vi "Update RefDAQ Parameters.vi"(0 "RefDAQParam":T1={"Full Frame Size"=0, "Ref Field of View"=0.0, "Ref Zoom"=0, "Ref_dwellTime"=0.0, "Ref X-pixels-per-line(Npxr)"=0, "Ref Y-lines-per-image(Npyr)"=0, "Ref Z-lines-per-image"=0, "Ignore Z lines"=0, "Ref Scan Cycles"=0, "Ref threshold XY"=0, "Ref threshold Z"=1, "Ref average XY"=1, "Ref Average  Z"=0, "Proportional_scale"=1.5999755859375, "Integral_scale"=2047.9375, "Proportional_scale Z"=1.5999755859375, "Integral_scale Z"=400.0, "Diff_threshold"=0.0, "Diff_threshold _z"=0.0, "Sliding Average"=FALSE, "Ref count reset enabled"=TRUE} caption="Reference frame DAQ setup" {"Proportional_scale Z" format="%#_15g"; "Ref average XY" min=1 max=64 step=1; "Diff_threshold" format="%#_15g"; "Diff_threshold _z" format="%#_15g"; "Proportional_scale" format="%#_15g"}, 11 "error in (no error)":errorcluster) -> (4 "Refnum out":T2, 15 "error out":errorcluster)   [LabVIEW 2020]
uses:
  RIG-SPECIFIC FILES/FPGA Refs/FPGA Ref.ctl
  Acquisition/Typedefs/Ref DAQ Param.ctl
  Typedefs/HW config states enum.ctl
  Global Variables/General Globals.vi
  Global Variables/gl_UI Ctrl Refs.vi
  <vilib>/Utility/error.llb/Error Cluster From Error Code.vi
  <vilib>/rvi/errors/niLvFpgaAdjustHostInterfaceError.vi
  <vilib>/rvi/interface/nirviReadWriteControl/nirviReadWriteControl.xnode
  NiFpgaLv.dll
  <vilib>/rvi/interface/Simulation/niFpgaSimulationCallBeginRW.vi
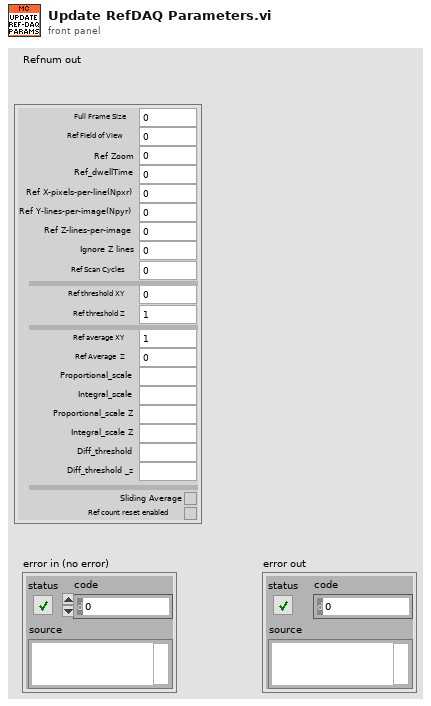
[diagram p1: front panel]
types:
  T1 = typedef "Ref DAQ Param.ctl" = cluster{"Full Frame Size":u16, "Ref Field of View":sgl, "Ref Zoom":i8, "Ref_dwellTime":sgl, "Ref X-pixels-per-line(Npxr)":i16, "Ref Y-lines-per-image(Npyr)":i16, "Ref Z-lines-per-image":i16, "Ignore Z lines":i16, "Ref Scan Cycles":i32, "Ref threshold XY":u16, "Ref threshold Z":u16, "Ref average XY":u16, "Ref Average  Z":u16, "Proportional_scale":fxp<+,16,2>, "Integral_scale":fxp<+/-,16,12>, "Proportional_scale Z":fxp<+,16,2>, "Integral_scale Z":fxp<+/-,16,12>, "Diff_threshold":fxp<+,16,2>, "Diff_threshold _z":fxp<+,16,2>, "Sliding Average":bool, "Ref count reset enabled":bool}
  T2 = typedef "FPGA Ref.ctl" = refnum<k20>
  T3 = typedef "HW config states enum.ctl" = enum16{"Load from file", "Save to file", "Save backup", "Write all", "Read all", "Write XY stage settings", "Write DAQ FPGA settings", "Write Control FPGA settings", "Write Phys Channels", "Write System Config", "Write HW Config", "Save System Config", "Save HW Config", "Clear", "Compare from file"}
  T4 = typedef "Hardware Configuration settings.ctl" = cluster{"Dev. PC":bool, "Swap XY on stage":bool, "No of AOD":u8, "MC Supported":bool, "Axial MC":bool, "Computer MAC address":string, "Externalise Triggers":bool, "Trigger HW config":T5, "DAQmx Chan":T6, "XY stage available":bool, "XY Stage":T7, "Z stage available":bool, "Z Stage config cluster":T8, "Encoder available":bool, "Encoder":T9, "VidRec available":bool, "Cam VidRec":T10, "Laser Power Control HW config":T11, "Laser 1 available":bool, "Laser 1 config cluster":T12, "Prechirper 1 available":bool, "Prechirper 1 config cluster":T13, "Control system.FPGA available?":bool, "Control Sys. HW config":T14, "DAQ FPGA HW Config":T15, "PMT Voltage Range":T18}
  T5 = typedef "Triggers HW config.ctl" = cluster{"Available Device List":i32, "Device Address":string}
  T6 = typedef "DAQmx physical channels cluster.ctl" = cluster{"Pockels AO":tag, "Hard shutter AO":tag, "PMT AOs":tag, "Galvo AOs":tag, "Power meter AI":tag}
  T7 = typedef "XY Stage config cluster.ctl" = cluster{"COM port":refnum<visa-resource-name>, "Baudrate":i32, "Type":string}
  T8 = typedef "Z Stage config cluster.ctl" = cluster{"COM port":refnum<visa-resource-name>, "Baudrate":i32, "Type":string}
  T9 = typedef "Encoder config cluster.ctl" = cluster{"IP address":string, "Port":u16, "Wheel radius (cm)":dbl, "Encoder Trigger":tag}
  T10 = typedef "Cam VidRec HW config setup cluster.ctl" = cluster{"DO flag-Video record":tag, "DO flag-Trial start":tag}
  T11 = typedef "Laser Power Control HW config.ctl" = cluster{"Laser Power Control":string, "Laser Power Modulation Control":enum16{"NI", "FPGA"}}
  T12 = typedef "Laser 1 config cluster.ctl" = cluster{"COM port":refnum<visa-resource-name>, "Baud Rate":i32, "Type":string}
  T13 = typedef "PreChirper 1 config cluster.ctl" = cluster{"Type":string, "Baud Rate":i32, "COM port":refnum<visa-resource-name>}
  T14 = typedef "Control Sys HW config cluster.ctl" = cluster{"Control system.FPGA Type":enum16{"Virtex 5", "Virtex 7"}, "Control system.Network adapter name":string, "Control system.MAC address":string, "Control system.Ethernet Port":u32, "Control system.Ethernet Port Opened":bool}
  T15 = typedef "DAQ FPGA HW config cluster.ctl" = cluster{"FGPA Ref":T2, "Target":T16, "input card type":T17}
  T16 = typedef "nirio_resource_hc.ctl" = tag
  T17 = typedef "FPGA input type AC-DC.ctl" = enum16{"AC Card", "DC Card"}
  T18 = typedef "PMT Voltage Range.ctl" = cluster{"PMT Voltage Lower Limit":dbl, "PMT Voltage Upper Limit":dbl}
  T19 = typedef "UI ctrl refs cluster.ctl" = cluster{"Top level VI path":path, "Top level VI ref":refnum<vi>, "User menu ref":refnum<k9>, "Sub Panel control":refnum<vi>, "Imaging Param Tab":refnum<vi>, "Occurrence-Start drivers":refnum<k4>, "Occurrence-Speed logging initialised":refnum<k4>, "Occurrence-XYZ stage initialised":refnum<k4>, "Exit button":refnum<vi>, "Status ind":refnum<vi>, "Set as origin":refnum<vi>, "Speed Logging":refnum<vi>, "Time Lapse":refnum<vi>, "Live Imaging":refnum<vi>, "AOL Z Stack":refnum<vi>, "Motor Z Stack":refnum<vi>, "Funct Acq button":refnum<vi>, "Hard Shutter":refnum<vi>, "Virtual Shutter":refnum<vi>, "Laser Power":refnum<vi>, "AOL Mode":refnum<vi>, "Frame Size":refnum<vi>, "Field of View":refnum<vi>, "Dwell Time":refnum<vi>, "Zoom":refnum<vi>, "AOL Z":refnum<vi>, "Objective":refnum<vi>, "Axis":refnum<vi>, "Paths & Names":refnum<vi>, "Experiment folder path (ind.)":refnum<vi>, "Last State (Ind.)":refnum<vi>, "Averages":refnum<vi>, "Angle (degrees)":refnum<vi>, "X centre":refnum<vi>, "Y centre":refnum<vi>, "Plane Mode":refnum<vi>, "# Planes":refnum<vi>, "Z Start":refnum<vi>, "Z Stop":refnum<vi>, "Z Step":refnum<vi>, "PMT 1":refnum<vi>, "PMT 2":refnum<vi>, "Stage XYZ Position":refnum<vi>, "Pockels@Z Start":refnum<vi>, "Pockels@Z Stop":refnum<vi>, "Obtain Z Start":refnum<vi>, "Obtain Z Stop":refnum<vi>, "Live stim.trig.period":refnum<vi>, "Live stim.trig.enable":refnum<vi>, "Movement Correction":refnum<vi>, "Load Reference Image":refnum<vi>, "XY Stage Move":refnum<vi>, "MovCor Cluster":refnum<vi>, "RefDAQParam":refnum<vi>, "Funct. Acq. Pockels Modulation":refnum<vi>, "Ref Laser Power":refnum<vi>, "Enable Video Recording":refnum<vi>, "Video Record-Live Imaging":refnum<vi>, "Video Record-Funct acq":refnum<vi>, "Reference Source":refnum<vi>, "AOL Z-stack Chirps Ready (ind)":refnum<vi>, "Target time between mov.cor. ref triggers (ms)":refnum<vi>, "Funct. Acq. Ref frame save":refnum<vi>, "Tracking button":refnum<vi>, "Show ref plots window":refnum<vi>, "Center freq ind (nm)":refnum<vi>, "Pickup mode (ind)":refnum<vi>, "Logging queue (ind)":refnum<vi>, "Back aperture power (ind.)":refnum<vi>, "Power after objective (ind.)":refnum<vi>, "Switch user":refnum<vi>, "Ls1 Conn. Status":refnum<vi>, "Ls1Tuning Status":refnum<vi>, "Ls1 Faults":refnum<vi>, "Ls1 Connection":refnum<vi>, "Ls1 Mode":refnum<vi>, "Ls1 POWER [mW]":refnum<vi>, "Ls1Shutter":refnum<vi>, "Ls1 Wavelength":refnum<vi>, "Ls1 Note":refnum<vi>, "Ls1 Confirm Wav":refnum<vi>, "Ls1 PreChrp Prism1":refnum<vi>, "Ls1 PreChrp Prism2":refnum<vi>, "Ls1 wav top Ind":refnum<vi>, "Ls1 power top Ind":refnum<vi>, "Ls1 Pump peak Hold":refnum<vi>, "Ls1 Status Ind":refnum<vi>, "Ls1 wav cancel":refnum<vi>, "Experiment Type":refnum<vi>, "Biology Information":refnum<vi>, "Camera recording status":refnum<vi>}
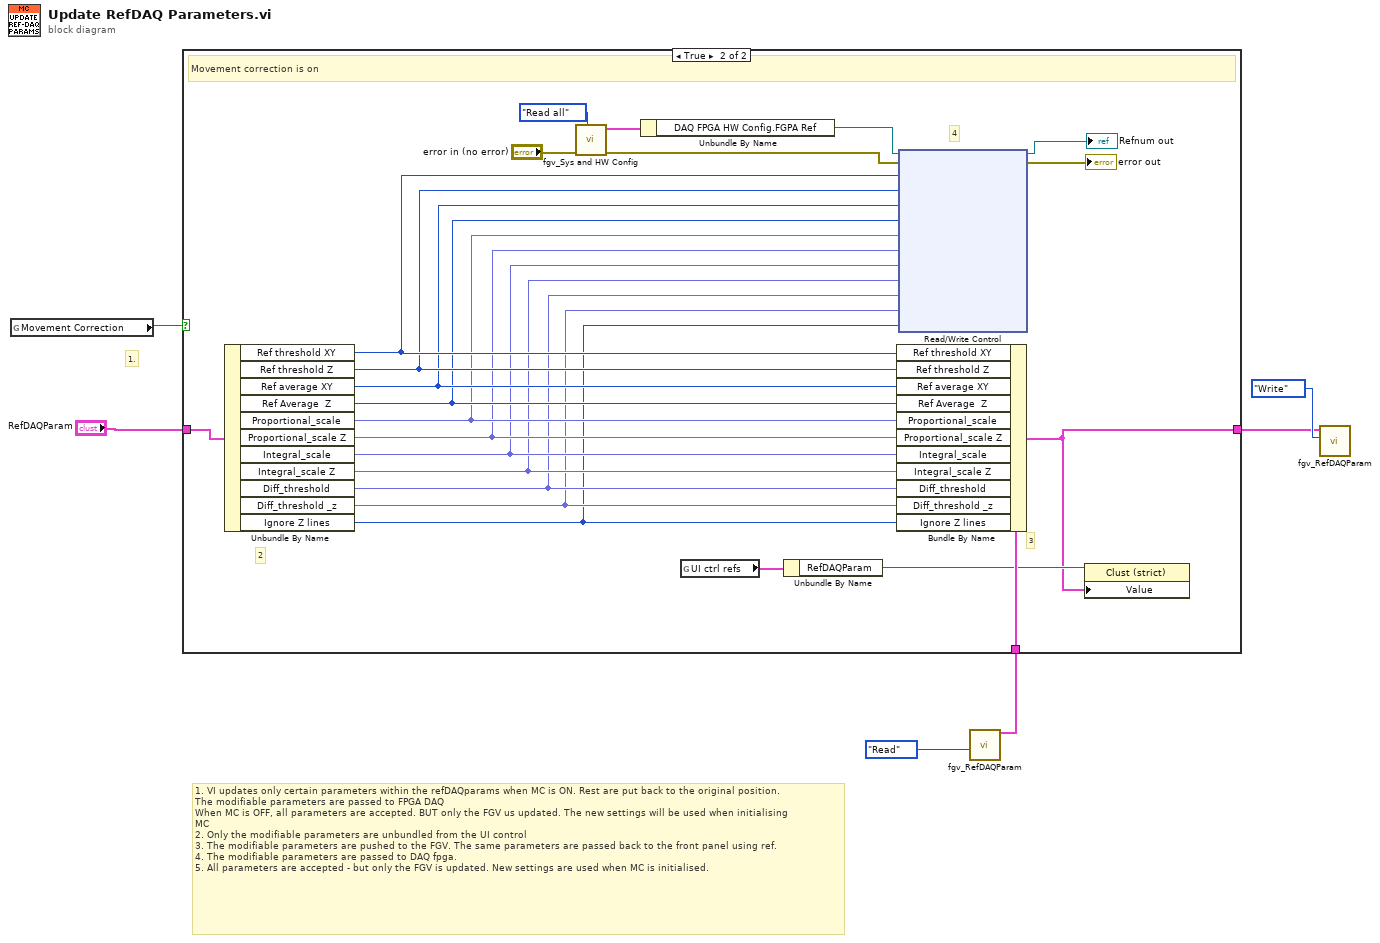
[diagram p0: block diagram]
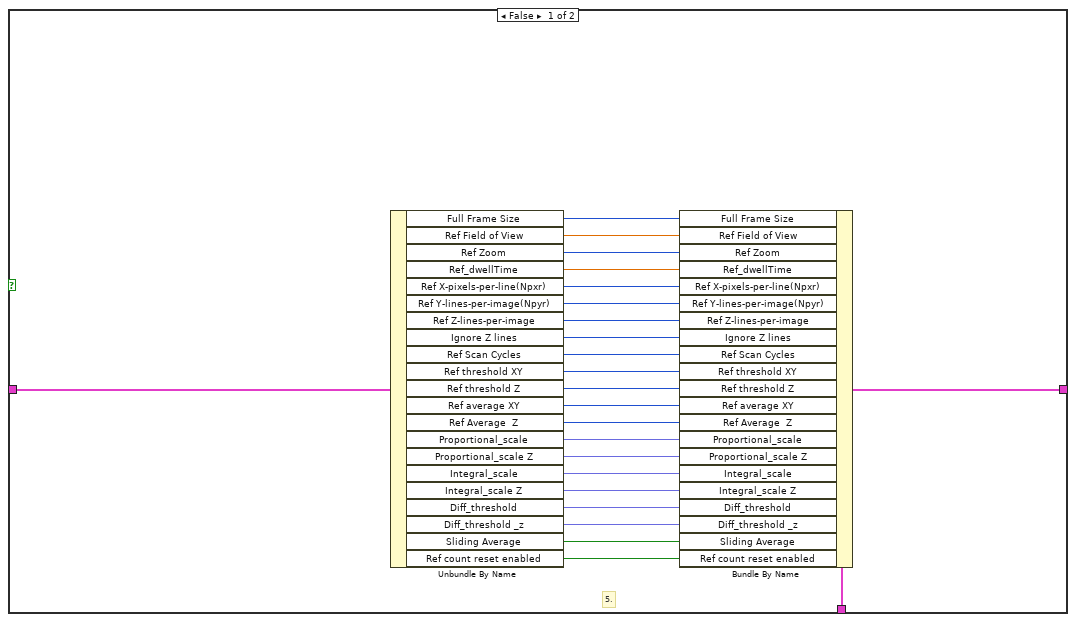
[diagram p2: hidden frame]
diagram:
  # "1. VI updates only certain parameters within the refDAQparams when MC is ON. Rest are put back to the original position.\nThe modifiable parameters are passed to FPGA DAQ\nWhen MC is OFF, all parameters are accepted. BUT only the FGV us updated. The new settings will be used when initialising \nMC\n2. Only the modifiable parameters are unbundled from the UI control\n3. The modifiable parameters are pushed to the FGV. The same parameters are passed back to the front panel using ref.\n4. The modifiable parameters are passed to DAQ fpga.\n5. All parameters are accepted - but only the FGV is updated. New settings are used when MC is initialised."
  # "1."
  n1 = global read "General Globals.vi" "Movement Correction"() -> (w6:bool)
  n2 = call "fgv_RefDAQParam.vi"("Function"=enum16{"Initialize", "Write", "Read"}."Read" ("Status")) -> ("RefDAQParam"=w3:T1)  [unwired: 9 in, 1 out]
  n3 = case shown="True" w6 {
    tunnel: "RefDAQParam" -> [w20 w46]
    tunnel: w3 -> [w8 w35]
    tunnel: [w7 w32] -> w1
    frame False {
      # "5."
      n4 = Unbundle By Name(w20) -> ("Full Frame Size"=w17:u16, "Ref Field of View"=w16:sgl, "Ref Zoom"=w15:i8, "Ref_dwellTime"=w14:sgl, "Ref X-pixels-per-line(Npxr)"=w13:i16, "Ref Y-lines-per-image(Npyr)"=w12:i16, "Ref Z-lines-per-image"=w11:i16, "Ignore Z lines"=w10:i16, "Ref Scan Cycles"=w9:i32, "Ref threshold XY"=w30:u16, "Ref threshold Z"=w29:u16, "Ref average XY"=w28:u16, "Ref Average  Z"=w27:u16, "Proportional_scale"=w26:fxp<+,16,2>, "Proportional_scale Z"=w25:fxp<+,16,2>, "Integral_scale"=w24:fxp<+/-,16,12>, "Integral_scale Z"=w23:fxp<+/-,16,12>, "Diff_threshold"=w22:fxp<+,16,2>, "Diff_threshold _z"=w21:fxp<+,16,2>, "Sliding Average"=w19:bool, "Ref count reset enabled"=w18:bool)
      n5 = Bundle By Name(cluster=w8, "Full Frame Size"=w17, "Ref Field of View"=w16, "Ref Zoom"=w15, "Ref_dwellTime"=w14, "Ref X-pixels-per-line(Npxr)"=w13, "Ref Y-lines-per-image(Npyr)"=w12, "Ref Z-lines-per-image"=w11, "Ignore Z lines"=w10, "Ref Scan Cycles"=w9, "Ref threshold XY"=w30, "Ref threshold Z"=w29, "Ref average XY"=w28, "Ref Average  Z"=w27, "Proportional_scale"=w26, "Proportional_scale Z"=w25, "Integral_scale"=w24, "Integral_scale Z"=w23, "Diff_threshold"=w22, "Diff_threshold _z"=w21, "Sliding Average"=w19, "Ref count reset enabled"=w18) -> (w7:T1)
    }
    frame True {
      # "4"
      # "3"
      # "2"
      # "Movement correction is on"
      n6 = Unbundle By Name(w46) -> ("Ref threshold XY"=w45:u16, "Ref threshold Z"=w44:u16, "Ref average XY"=w43:u16, "Ref Average  Z"=w42:u16, "Proportional_scale"=w41:fxp<+,16,2>, "Proportional_scale Z"=w40:fxp<+,16,2>, "Integral_scale"=w39:fxp<+/-,16,12>, "Integral_scale Z"=w38:fxp<+/-,16,12>, "Diff_threshold"=w37:fxp<+,16,2>, "Diff_threshold _z"=w36:fxp<+,16,2>, "Ignore Z lines"=w31:i16)
      n7 = call "fgv_Sys and HW Config.vi"("Function"=HW_config_states_enum."Read all", "error in (no error)"="error in (no error)") -> ("error out"=w50:errorcluster, "Hardware Configuration OUT"=w52:T4)  [unwired: 7 in, 1 out]
      n8 = Unbundle By Name(w52) -> ("DAQ FPGA HW Config.FGPA Ref"=w51:T2)
      n9 = global read "gl_UI Ctrl Refs.vi" "UI ctrl refs"() -> (w34:T19)
      n10 = Unbundle By Name(w34) -> ("RefDAQParam"=w33:refnum<vi>)
      n11 = Bundle By Name(cluster=w35, "Ref threshold XY"=w45, "Ref threshold Z"=w44, "Ref average XY"=w43, "Ref Average  Z"=w42, "Proportional_scale"=w41, "Proportional_scale Z"=w40, "Integral_scale"=w39, "Integral_scale Z"=w38, "Diff_threshold"=w37, "Diff_threshold _z"=w36, "Ignore Z lines"=w31) -> (w32:T1)
      n12 = xnode ("Read/Write Control")("FPGA VI Reference In"=w51, "error in"=w50, "threshold_xy"=w45, "threshold_z"=w44, "Average"=w43, "Average Z"=w42, "proportioanl_scale"=w41, "proportioanl_scale _z"=w40, "Integral_scale_ind"=w39, "Integral_scale z"=w38, "diff_thresh"=w37, "diff_thresh_z"=w36, "ignore_z_lines"=w31) -> ("FPGA VI Reference Out"=→"Refnum out":T2, "error out"=→"error out":errorcluster)
      n13 = property class="Clust (strict)"(reference=w33, "Value"=w32) -> ()  [unwired: 1 in, 2 out]
    }
  }
  n14 = call "fgv_RefDAQParam.vi"("Function"=enum16{"Initialize", "Write", "Read"}."Write" ("Status"), "RefDAQParam in"=w1) -> ()  [unwired: 8 in, 2 out]
